vi "TcpServer.vi"() -> ()   [LabVIEW 2021]
doc: "Demonstrates how to set up a basic TCP connection, send data to the specified port once a connection has been established, and terminate the connection once the data has been sent. This VI is designed to stop if the TCP connection is terminated. The data sent in this example is an array of random numbers."
panel:
  out "?":bool
  out "clientReady":bool
  out "?":dbl format="%%%.1f"
  out "progress":dbl(slide) scale=0.0..100.0
  in  "?":bool
  in  "partitionSize":i64=50000 min=1 max=100000000 step=1
  in  "?":path
  in  "Client Closed":string="The client VI closed the connection."
  # "click here to choose a file， \nthen click ok to start  send"
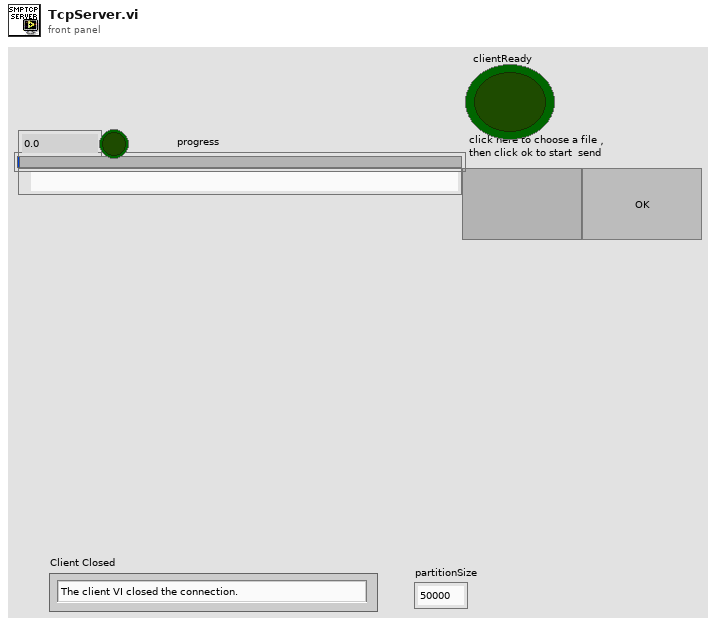
[diagram p1: front panel]
types:
  T1 = enum16{"open", "replace", "create", "open or create", "replace or create", "replace or create with confirmation"}
  T2 = enum16{"big-endian, network order", "native, host order", "little-endian"}
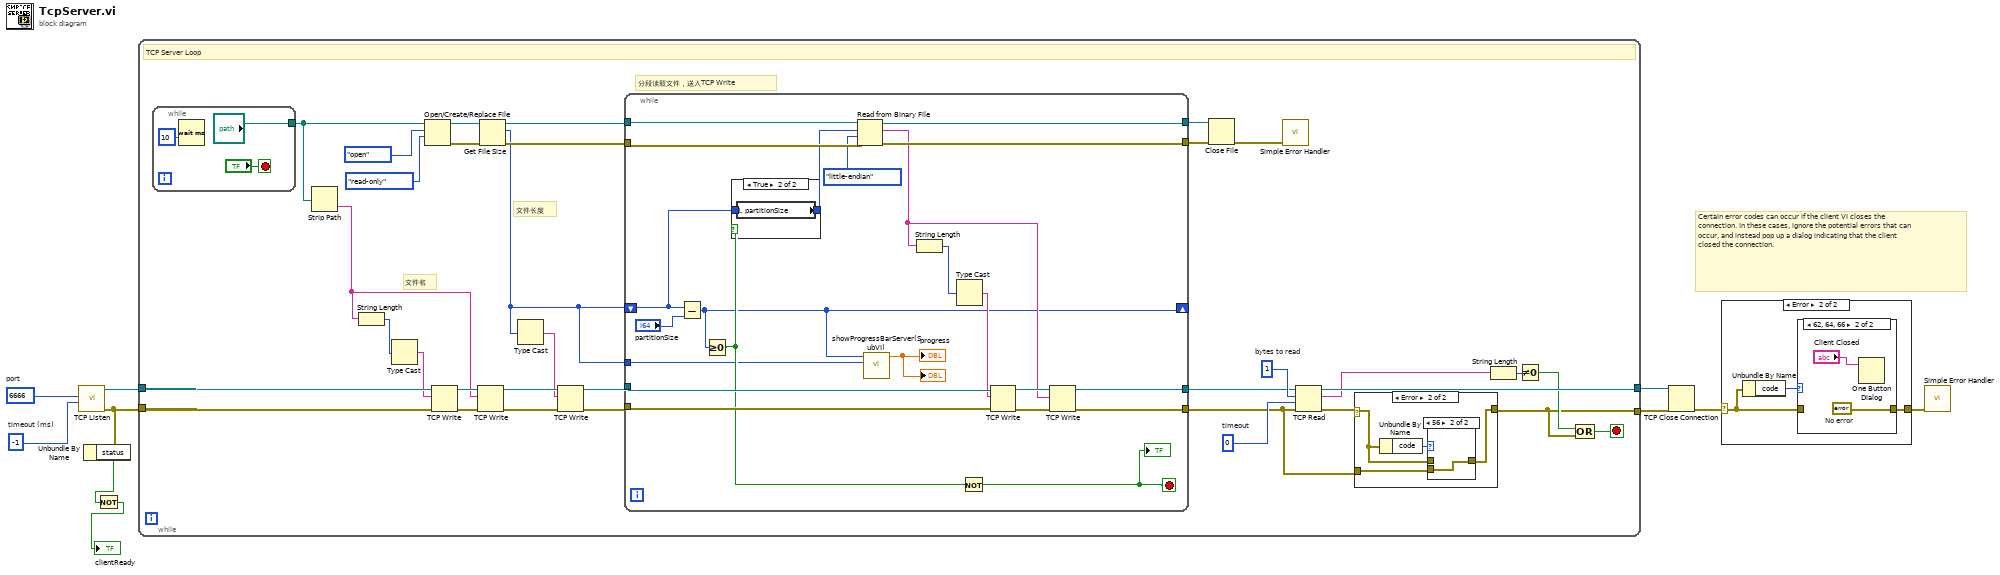
[diagram p0: block diagram]
diagram:
  w4 = u16 6666  # port
  w5 = -1  # timeout (ms)
  # "Certain error codes can occur if the client VI closes the connection. In these cases, ignore the potential errors that can occur, and instead pop up a dialog indicating that the client closed the connection."
  n1 = call <vilib>:"TCP Listen.vi"("timeout ms (wait forever: -1)"=w5, "port"=w4) -> ("error out"=w3:errorcluster, "connection ID"=w6:refnum<k5>)  [unwired: 5 in, 3 out]
  n2 = Unbundle By Name(w3) -> ("status"=w1:bool)
  n3 = Not(x=w1) -> (.not. x?=→"clientReady":bool)
  n4 = while {
    tunnel: [w36] -> w9
    tunnel: [w42] -> w10
    tunnel: w6 -> [w34]
    tunnel: w3 -> [w35]
    stop <- w44 stop-if-true
    w41 = 0  # timeout
    w43 = 1  # bytes to read
    # "分段读取文件，送入TCP Write"
    # "文件长度"
    # "文件名"
    # "TCP Server Loop"
    n5 = while {
      tunnel: ["?"] -> w14
      stop <- "?" stop-if-true
      n6 = Wait (ms)(milliseconds to wait=u32 10) -> ()  [unwired: 1 out]
    }
    n7 = Strip Path(path=w14) -> (name=w30:string)  [unwired: 1 out]
    n8 = String Length(string=w30) -> (length=w15:i32)
    n9 = Type Cast(x=w15) -> (*(type *) &x=w31:string)  [unwired: 1 in]
    n10 = Open/Create/Replace File(file path (use dialog)=w14, operation (0:open)=T1."open", access (0:read/write)=enum16{"read/write", "read-only", "write-only"}."read-only") -> (refnum out=w25:refnum<file>, error out=w24:errorcluster)  [unwired: 3 in, 1 out]
    n11 = TCP Write(connection ID=w34, data in=w31, error in (no error)=w35) -> (connection ID out=w33:refnum<k5>, error out=w32:errorcluster)  [unwired: 1 in, 1 out]
    n12 = TCP Write(connection ID=w33, data in=w30, error in (no error)=w32) -> (connection ID out=w29:refnum<k5>, error out=w28:errorcluster)  [unwired: 1 in, 1 out]
    n13 = Get File Size(file=w25, error in=w24) -> (refnum out=w22:refnum<file>, size (in bytes)=w12:i64, 0:w19:errorcluster)
    n14 = Type Cast(x=w12) -> (*(type *) &x=w23:string)  [unwired: 1 in]
    n15 = TCP Write(connection ID=w29, data in=w23, error in (no error)=w28) -> (connection ID out=w21:refnum<k5>, error out=w20:errorcluster)  [unwired: 1 in, 1 out]
    n16 = while {
      tunnel: w22 -> [w63]
      tunnel: w21 -> [w69]
      tunnel: w20 -> [w56]
      tunnel: w19 -> [w64]
      tunnel: [w53] -> w13
      tunnel: [w67] -> w18
      tunnel: [w66] -> w17
      tunnel: [w65] -> w16
      shift-right: [w51] -> _
      shift-left: w12 -> [w57]
      tunnel: w12 -> [w50]
      stop <- w48 stop-if-true
      n17 = Subtract(x=w57, y="partitionSize") -> (x-y=w51:i64)
      n18 = Greater Or Equal To 0?(x=w51) -> (x >= 0?=w52:bool)
      n19 = case shown="True" w52 {
        tunnel: [w70 w71] -> w58
        tunnel: w57 -> [w70 _]
        frame False {
        }
        frame True {
          n20 = local read "partitionSize"() -> (w71:i64)
        }
      }
      n21 = Read from Binary File(8:w64, 9:T2."little-endian" ("byte order (0:big-endian, network order)"), 10:w58, 11:w63) -> (0:w66:errorcluster, 2:w59:string, 3:w65:refnum<file>)  [unwired: 2 in, 1 out]
      n22 = call "showProgressBarServer(SubVI).vi"("file size"=w50, "to be transmitted"=w51) -> ("progress bar"=→"progress" →"?":dbl)  [unwired: 9 in]
      n23 = String Length(string=w59) -> (length=w61:i32)
      n24 = Type Cast(x=w61) -> (*(type *) &x=w60:string)  [unwired: 1 in]
      n25 = Not(x=w52) -> (.not. x?=w48:bool)
      "?" <- w48
      n26 = TCP Write(connection ID=w69, data in=w60, error in (no error)=w56) -> (connection ID out=w68:refnum<k5>, error out=w54:errorcluster)  [unwired: 2 out]
      n27 = TCP Write(connection ID=w68, data in=w59, error in (no error)=w54) -> (connection ID out=w67:refnum<k5>, error out=w53:errorcluster)  [unwired: 2 out]
    }
    n28 = Close File(refnum=w16, error in=w17) -> (error out=w11:errorcluster)  [unwired: 1 out]
    n29 = call <vilib>:"Simple Error Handler.vi"("error in (no error)"=w11) -> ()  [unwired: 4 in, 5 out]
    n30 = TCP Read(connection ID=w18, bytes to read=w43, error in (no error)=w13, 9:w41) -> (connection ID out=w42:refnum<k5>, data out=w39:string, error out=w37:errorcluster)  [unwired: 1 out]
    n31 = case shown="Error" w37 {
      selector: w37 -> [w72 w75]
      tunnel: [w72 w73] -> w36
      tunnel: w13 -> [_ w74]
      frame No Error {
      }
      frame Error {
        n32 = Unbundle By Name(w75) -> ("code"=w76:i32)
        n33 = case shown="56" w76 {
          tunnel: w75 -> [w77 _]
          tunnel: w74 -> [_ w78]
          tunnel: [w77 w78] -> w73
          frame Default {
          }
          frame 56 {
          }
        }
      }
    }
    n34 = String Length(string=w39) -> (length=w40:i32)
    n35 = Not Equal To 0?(x=w40) -> (x != 0?=w38:bool)
    n36 = Compound Arithmetic op=OR(w38, w36) -> (w44:bool)
  }
  n37 = TCP Close Connection(connection ID=w10, error in (no error)=w9) -> (error out=w8:errorcluster)  [unwired: 2 out]
  n38 = case shown="Error" w8 {
    selector: w8 -> [w79 w81]
    tunnel: [w79 w80] -> w7
    frame No Error {
    }
    frame Error {
      n39 = Unbundle By Name(w81) -> ("code"=w82:i32)
      n40 = case shown="62, 64, 66" w82 {
        tunnel: w81 -> [w83 _]
        tunnel: [w83 w85] -> w80
        frame Default {
        }
        frame 62, 64, 66 {
          w85 = errorcluster {"status"=FALSE, "code"=0, "source"=""}  # No error
          n41 = One Button Dialog(message="Client Closed") -> ()  [unwired: 1 in, 1 out]
        }
      }
    }
  }
  n42 = call <vilib>:"Simple Error Handler.vi"("error in (no error)"=w7) -> ()  [unwired: 1 in, 8 out]
